vi "create_queue_temp.vi"(11 "Value":dbl) -> (2 "Current Queue":dbl[](array[numeric]), 3 "Boolean":bool)   [LabVIEW 2015]
uses:
  <vilib>/ptbypt/NI_PtbyPt.lvlib
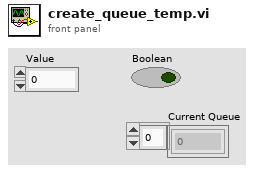
[diagram p1: front panel]
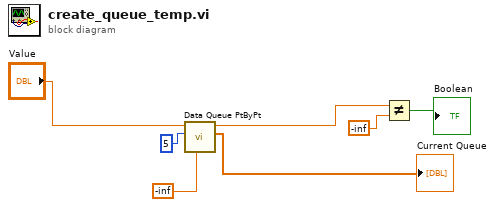
[diagram p0: block diagram]
diagram:
  n1 = call <vilib>:"Data Queue PtByPt.vi"("initial queue element"=-inf, "sample length"=5, "input data point"="Value") -> ("Current Queue"=→"Current Queue":dbl[], "eliminated element"=w4:dbl)  [unwired: 4 in, 3 out]
  n2 = Not Equal?(x=w4, y=-inf) -> (x != y?=→"Boolean":bool)
